vi "AddClassToProject.vi"(8 "error in (no error)":errorcluster, 11 "baseClass in":refnum<class "baseClass.lvclass">) -> (0 "error out":errorcluster, 3 "baseClass out":refnum<class "baseClass.lvclass">)   [LabVIEW 2013, in "baseClass.lvclass"]
uses:
  baseClass.lvclass
  ProjectHandler/RefNums.vi
  ProjectHandler.lvlib
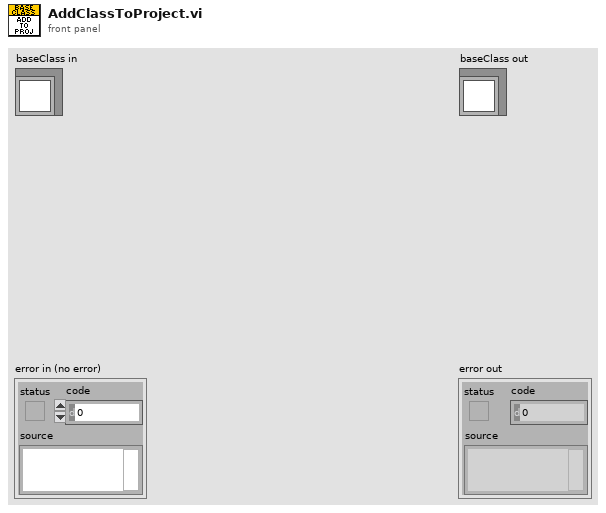
[diagram p1: front panel]
types:
  T1 = cluster{"App":refnum<vi>, "Project":refnum<vi>, "My Computer":refnum<vi>}
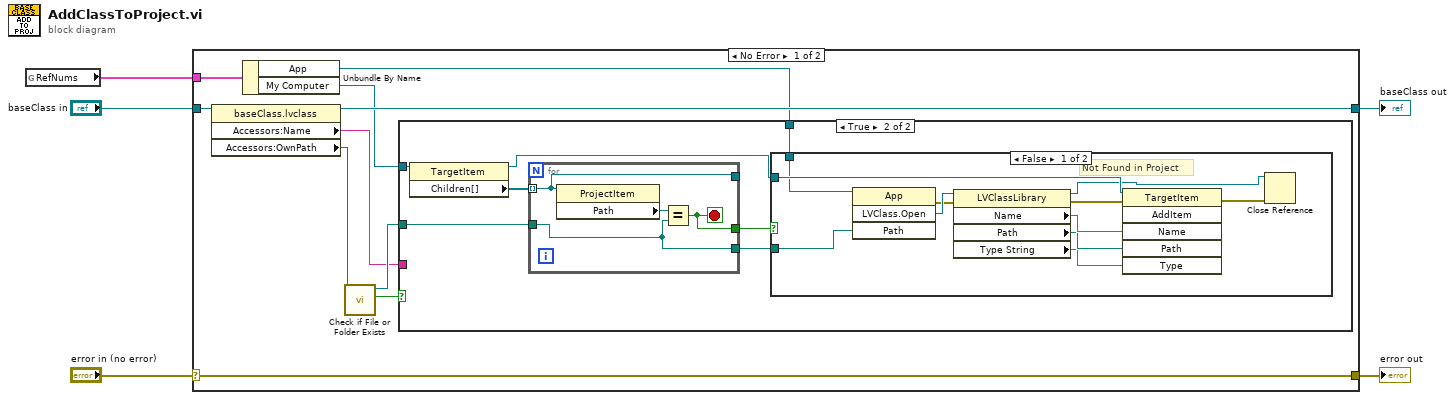
[diagram p0: block diagram]
diagram:
  n1 = global read "RefNums.vi" "RefNums"() -> (w1:T1)
  n2 = case shown="No Error" "error in (no error)" {
    selector: "error in (no error)" -> [w14 w39]
    tunnel: [w14 w39] -> w4
    tunnel: [w13 w38] -> w2
    tunnel: "baseClass in" -> [w15 w38]
    tunnel: w1 -> [w12 _]
    frame No Error {
      n3 = property class="baseClass.lvclass"(reference=w15) -> (reference out=w13:refnum<class "baseClass.lvclass">, "Accessors:Name"=w7:string, "Accessors:OwnPath"=w11:path)  [unwired: 1 in, 1 out]
      n4 = Unbundle By Name(w12) -> ("App"=w6:refnum<vi>, "My Computer"=w10:refnum<vi>)
      n5 = call <vilib>:"Check if File or Folder Exists.vi"("path"=w11) -> ("file or folder exists?"=w8:bool, "dup path"=w9:path)  [unwired: 8 in, 1 out]
      n6 = case shown="True" w8 {
        tunnel: w10 -> [_ w22]
        tunnel: w9 -> [_ w20]
        tunnel: w7 -> [_ _]
        tunnel: w6 -> [_ w16]
        frame False {
        }
        frame True {
          n7 = property class="TargetItem"(reference=w22) -> (reference out=w19:refnum<vi>, "Children[]"=w21:refnum<vi>[])  [unwired: 1 in, 1 out]
          n8 = for {
            tunnel: w21 -> [w34] mode=indexing
            tunnel: w20 -> [w35]
            tunnel: [w36] -> w18
            tunnel: [w35] -> w17
            tunnel: [w34] -> _
            stop <- w36 stop-if-true
            n9 = property class="ProjectItem"(reference=w34) -> ("Path"=w37:path)  [unwired: 1 in, 2 out]
            n10 = Equal?(x=w37, y=w35) -> (x = y?=w36:bool)
          }
          n11 = case shown="False" w18 {
            tunnel: w19 -> [w33 _]
            tunnel: w17 -> [w31 _]
            tunnel: w16 -> [w32 _]
            frame False {
              # "Not Found in Project"
              n12 = invoke class="App" method="LVClass.Open"(reference=w32, "Path"=w31) -> (error out=w26:errorcluster, "LVClass.Open"=w30:refnum<vi>)  [unwired: 2 in, 2 out]
              n13 = property class="LVClassLibrary"(reference=w30, error in=w26) -> (reference out=w24:refnum<vi>, error out=w25:errorcluster, "Name"=w29:string, "Path"=w28:path, "Type String"=w27:string)
              n14 = invoke class="TargetItem" method="AddItem"(reference=w33, error in=w25, "Name"=w29, "Path"=w28, "Type"=w27) -> (error out=w23:errorcluster)  [unwired: 1 in, 5 out]
              n15 = Close Reference(reference=w24, error in (no error)=w23) -> ()  [unwired: 1 out]
            }
            frame True {
            }
          }
        }
      }
    }
    frame Error {
    }
  }
  "error out" <- w4
  "baseClass out" <- w2
